vi "Init Events.vi"(8 "error in (no error)":errorcluster, 11 "DiscoveryService in":refnum<class "DiscoveryService.lvclass">) -> (0 "error out":errorcluster, 3 "DiscoveryService out":refnum<class "DiscoveryService.lvclass">)   [LabVIEW 2020, in "Vecto.lvlib" / "DiscoveryService.lvclass"]
uses:
  DiscoveryService.lvclass
  Incoming Events.ctl
  Update Service Data.ctl
  proto/Service/Data.ctl
  proto/ServiceType/Enumeration.ctl
  DiscoveryService.lvclass/DiscoveryService.ctl
  proto/ServiceType/ServiceType.lvlib
  proto/Service/Service.lvlib
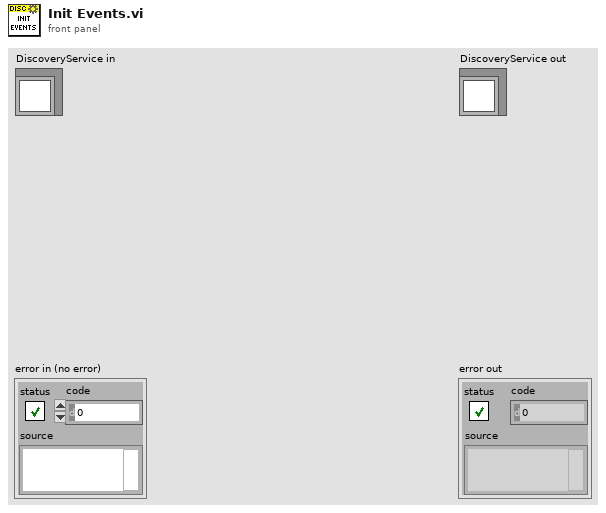
[diagram p1: front panel]
types:
  T1 = typedef "ServiceType.lvlib/Enumeration.ctl" = enum16{"SERVICETYPE_UNKNOWN", "SERVICETYPE_TCPSERVER", "SERVICETYPE_HTTPSERVER"}
  T2 = typedef "Vecto.lvlib/DiscoveryService.lvclass/Update Service Data.ctl" = cluster{"Service":T3}
  T3 = typedef "Service.lvlib/Data.ctl" = cluster{"type":T1, "port":i32}
  T4 = typedef "Vecto.lvlib/DiscoveryService.lvclass/Incoming Events.ctl" = cluster{"Close":refnum<user-event>, "Update Service":refnum<user-event>, "Update Status":refnum<user-event>, "Remove Service":refnum<user-event>}
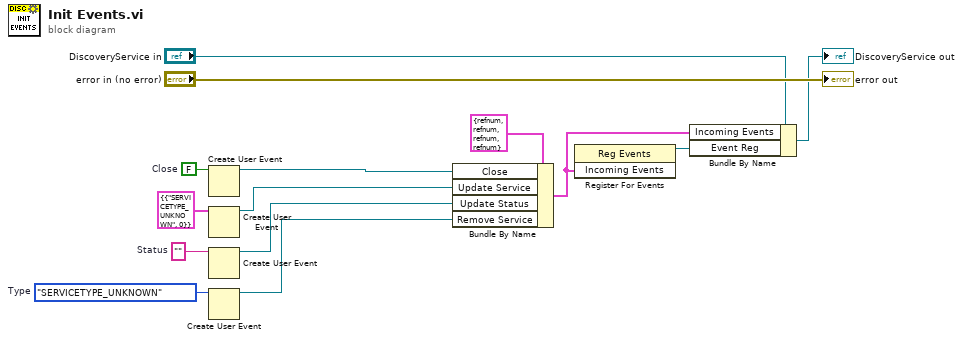
[diagram p0: block diagram]
diagram:
  w2 = Enumeration."SERVICETYPE_UNKNOWN"  # Type
  w4 = ""  # Status
  w13 = FALSE  # Close
  n1 = Create User Event(user event datatype=w13) -> (user event=w11:refnum<user-event>)  [unwired: 1 in, 1 out]
  n2 = Create User Event(user event datatype=T2 {"Service"={"type"=enum."SERVICETYPE_UNKNOWN", "port"=0}} ("Update Service Data")) -> (user event=w5:refnum<user-event>)  [unwired: 1 in, 1 out]
  n3 = Create User Event(user event datatype=w4) -> (user event=w3:refnum<user-event>)  [unwired: 1 in, 1 out]
  n4 = Create User Event(user event datatype=w2) -> (user event=w1:refnum<user-event>)  [unwired: 1 in, 1 out]
  n5 = Bundle By Name(cluster=T4 {"Close"=refnum, "Update Service"=refnum, "Update Status"=refnum, "Remove Service"=refnum} ("Incoming Events"), "Close"=w11, "Update Service"=w5, "Update Status"=w3, "Remove Service"=w1) -> (w9:T4)
  n6 = register-events(w9) -> (reference out=w8:refnum<event-registration>)  [unwired: 2 in, 1 out]
  n7 = Bundle By Name(cluster="DiscoveryService in", "Incoming Events"=w9, "Event Reg"=w8) -> (→"DiscoveryService out":refnum<class "DiscoveryService.lvclass">)
  "error out" <- "error in (no error)"
